vi "ex41.vi"(10 "Data":string, 11 "Data 2":string) -> ()   [LabVIEW 2019]
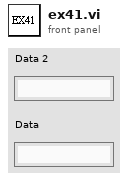
[diagram p1: front panel]
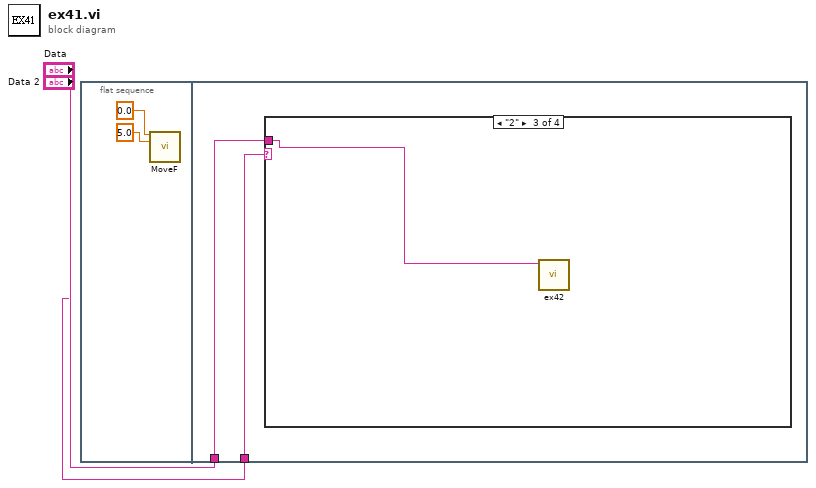
[diagram p0: block diagram]
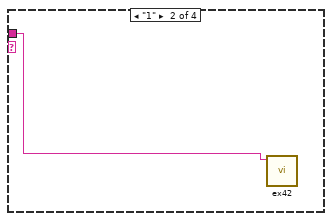
[diagram p3: hidden frame]
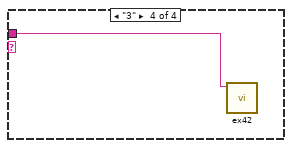
[diagram p4: hidden frame]
diagram:
  n1 = flat-sequence {
    tunnel: "Data 2" -> [w6]
    tunnel: "Data" -> [w5]
    frame #0 {
      n2 = call "MoveF.vi"("X"=0.0, "Y"=5.0) -> ()  [unwired: 13 in, 1 out]
    }
    frame #1 {
      n3 = case shown="\"2\"" w6 {
        tunnel: w5 -> [_ w7 w8 w9]
        frame "0", Default {
        }
        frame "1" {
          n4 = call "ex42.vi"("Data"=w7) -> ()  [unwired: 11 in]
        }
        frame "2" {
          n5 = call "ex42.vi"("Data"=w8) -> ()  [unwired: 11 in]
        }
        frame "3" {
          n6 = call "ex42.vi"("Data"=w9) -> ()  [unwired: 11 in]
        }
      }
    }
  }
